vi "LedColor.vi"(0 "Boolean in":refnum<vi>, 5 "Color Box":u32, 11 "error in (no error)":errorcluster) -> (15 "error out":errorcluster)   [LabVIEW 2011]
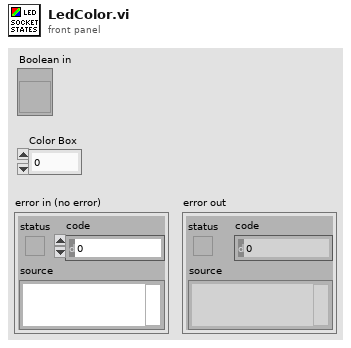
[diagram p1: front panel]
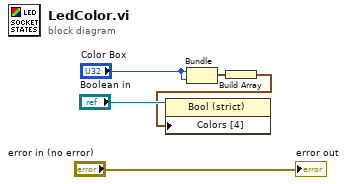
[diagram p0: block diagram]
diagram:
  n1 = Bundle("Color Box"="Color Box", "Color Box"="Color Box") -> (w3:cluster{"Color Box":u32, "Color Box":u32})  [unwired: 1 in]
  n2 = Build Array(w3) -> (w2:cluster{"Color Box":u32, "Color Box":u32}[])
  n3 = property on="Property Node" class="Bool (strict)"(reference="Boolean in", "Colors [4]"=w2) -> ()  [unwired: 1 in, 2 out]
  "error out" <- "error in (no error)"
